vi "Save Camera Status.vi"(8 "Action In":T1, 10 "Display State In":T2={"Pause"=FALSE, "Camera"={"Position"={"X"=0.0, "Y"=0.0, "Z"=4.0}, "Target"={"X"=0.0, "Y"=0.0, "Z"=0.0}, "Up Direction"={"X"=0.0, "Y"=1.0, "Z"=0.0}}, "Background Color"={"Red"=0.0, "Green"=0.0, "Blue"=0.0, "Alpha"=0.0}, "3DRefnum"=refnum}, 11 "ModelView Matrix":sgl[][](array[numeric])) -> (0 "Action Out":T1, 2 "Display State Out":T2={"Pause"=FALSE, "Camera"={"Position"={"X"=0.0, "Y"=0.0, "Z"=4.0}, "Target"={"X"=0.0, "Y"=0.0, "Z"=0.0}, "Up Direction"={"X"=0.0, "Y"=1.0, "Z"=0.0}}, "Background Color"={"Red"=0.0, "Green"=0.0, "Blue"=0.0, "Alpha"=0.0}, "3DRefnum"=refnum})   [LabVIEW 2017, in "Simulator Display.xctl"]
uses:
  <vilib>/robotics/Controls/Simulator Display/Simulator Display.xctl
  <vilib>/robotics/Controls/Simulator Display/State.ctl
  <vilib>/Utility/miscctls.llb/LVRGBAColorTypeDef.ctl
  <vilib>/_xctls/Action.ctl
  <vilib>/Analysis/baseanly.llb/A x Vector.vi
  <vilib>/Analysis/baseanly.llb/Real Inverse Matrix.vi
  <vilib>/Analysis/NI_AALBase.lvlib
  <vilib>/robotics/Kinematics/NI_Kinematics.lvlib
  <vilib>/_xctls/XControlSupport.lvlib
panel:
  out "Up":cluster{"X":dbl, "Y":dbl, "Z":dbl}
  out "Target":cluster{"X":dbl, "Y":dbl, "Z":dbl}
  out "Position":cluster{"X":dbl, "Y":dbl, "Z":dbl}
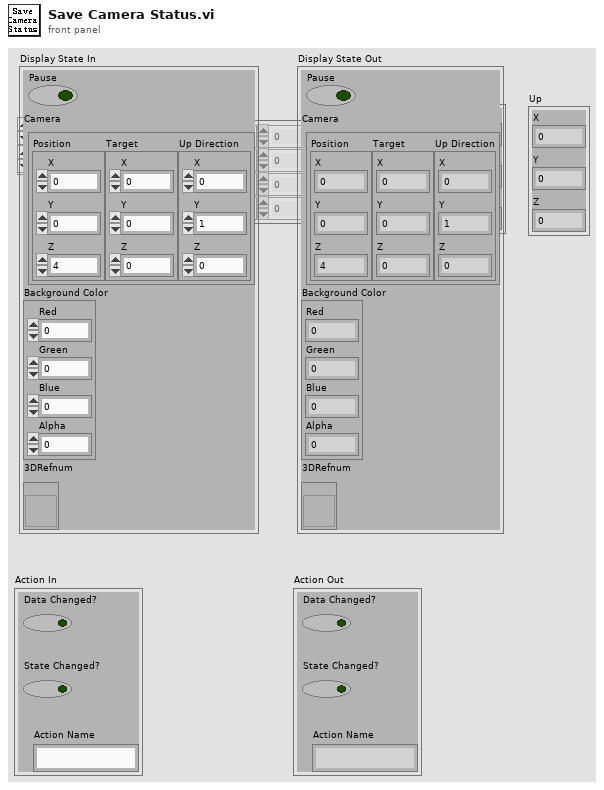
[diagram p1: front panel]
types:
  T1 = typedef "XControlSupport.lvlib/Action.ctl" = cluster{"Data Changed?":bool, "State Changed?":bool, "Action Name":string}
  T2 = typedef "Simulator Display.xctl/State.ctl" = cluster{"Pause":bool, "Camera":cluster{"Position":cluster{"X":dbl, "Y":dbl, "Z":dbl}, "Target":cluster{"X":dbl, "Y":dbl, "Z":dbl}, "Up Direction":cluster{"X":dbl, "Y":dbl, "Z":dbl}}, "Background Color":T3, "3DRefnum":refnum<vi>}
  T3 = typedef "LVRGBAColorTypeDef.ctl" = cluster{"Red":sgl, "Green":sgl, "Blue":sgl, "Alpha":sgl}
  T4 = typedef "NI_Matrix.lvlib/RealMatrix.ctl" = dbl[][]
  T5 = cluster{"A x Vector[0]":dbl, "A x Vector[1]":dbl, "A x Vector[2]":dbl}
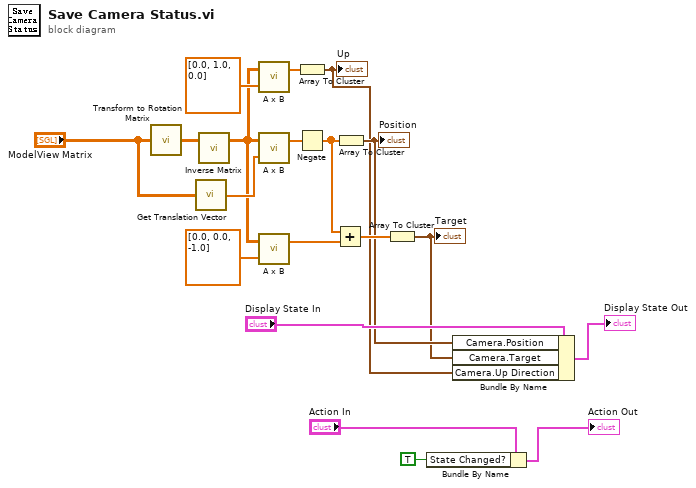
[diagram p0: block diagram]
diagram:
  n1 = call <vilib>:"Transform to Rotation Matrix.vi"("transform"="ModelView Matrix") -> ("rotation matrix"=w17:T4)
  n2 = call <vilib>:"Get Translation Vector.vi"("transform"="ModelView Matrix") -> ("translation vector"=w18:dbl[])
  n3 = call-poly <vilib>:"Inverse Matrix.vi"("Input Matrix"=w17) -> ("Inverse Matrix"=w14:T4)  [unwired: 1 in, 1 out]
  n4 = call-poly <vilib>:"A x B.vi"("Vector"=sgl[] [0.0, 1.0, 0.0], "A"=w14) -> ("A x Vector"=w13:dbl[])  [unwired: 1 out]
  n5 = call-poly <vilib>:"A x B.vi"("Vector"=w18, "A"=w14) -> ("A x Vector"=w12:dbl[])  [unwired: 1 out]
  n6 = call-poly <vilib>:"A x B.vi"("Vector"=sgl[] [0.0, 0.0, -1.0], "A"=w14) -> ("A x Vector"=w10:dbl[])  [unwired: 1 out]
  n7 = Array To Cluster(array=w13) -> (cluster=w5:T5)
  "Up" <- w5
  n8 = Negate(x=w12) -> (-x=w11:dbl[])
  n9 = Add(x=w11, y=w10) -> (x+y=w9:dbl[])
  n10 = Array To Cluster(array=w11) -> (cluster=w7:cluster{"[0]":dbl, "[1]":dbl, "[2]":dbl})
  "Position" <- w7
  n11 = Array To Cluster(array=w9) -> (cluster=w6:cluster{"[0]":dbl, "[1]":dbl, "[2]":dbl})
  "Target" <- w6
  n12 = Bundle By Name(cluster="Action In", "State Changed?"=TRUE) -> (→"Action Out":T1)
  n13 = Bundle By Name(cluster="Display State In", "Camera.Position"=w7, "Camera.Target"=w6, "Camera.Up Direction"=w5) -> (→"Display State Out":T2)
